vi "can_decoder2.vi"() -> ()   [LabVIEW 2015]
panel:
  out "tmp":dbl
  out "Waveform Chart 2":dynamicdata(graph)
  out "rate":dbl[](array[numeric]) format="%.2f"
  out "steering_torque":dbl format="%.2f"
  out "steering_angle":dbl format="%.2f"
  in  "IDs":u32[](array[numeric])=[0] format="%03x"
  in  "col size":i32
  in  "col idx":i32
  in  "ID":u32 format="%03x"
  out "Waveform Chart":dynamicdata(graph)
  in  "sortbyID":bool
  in  "clear":bool
  in  "sortbytime":bool
  out "can_log":u32[][](array[numeric]) format="%02x"
  out "error out":errorcluster
  # "Steering angle"
  # "Steering torque"
  # "RATE?"
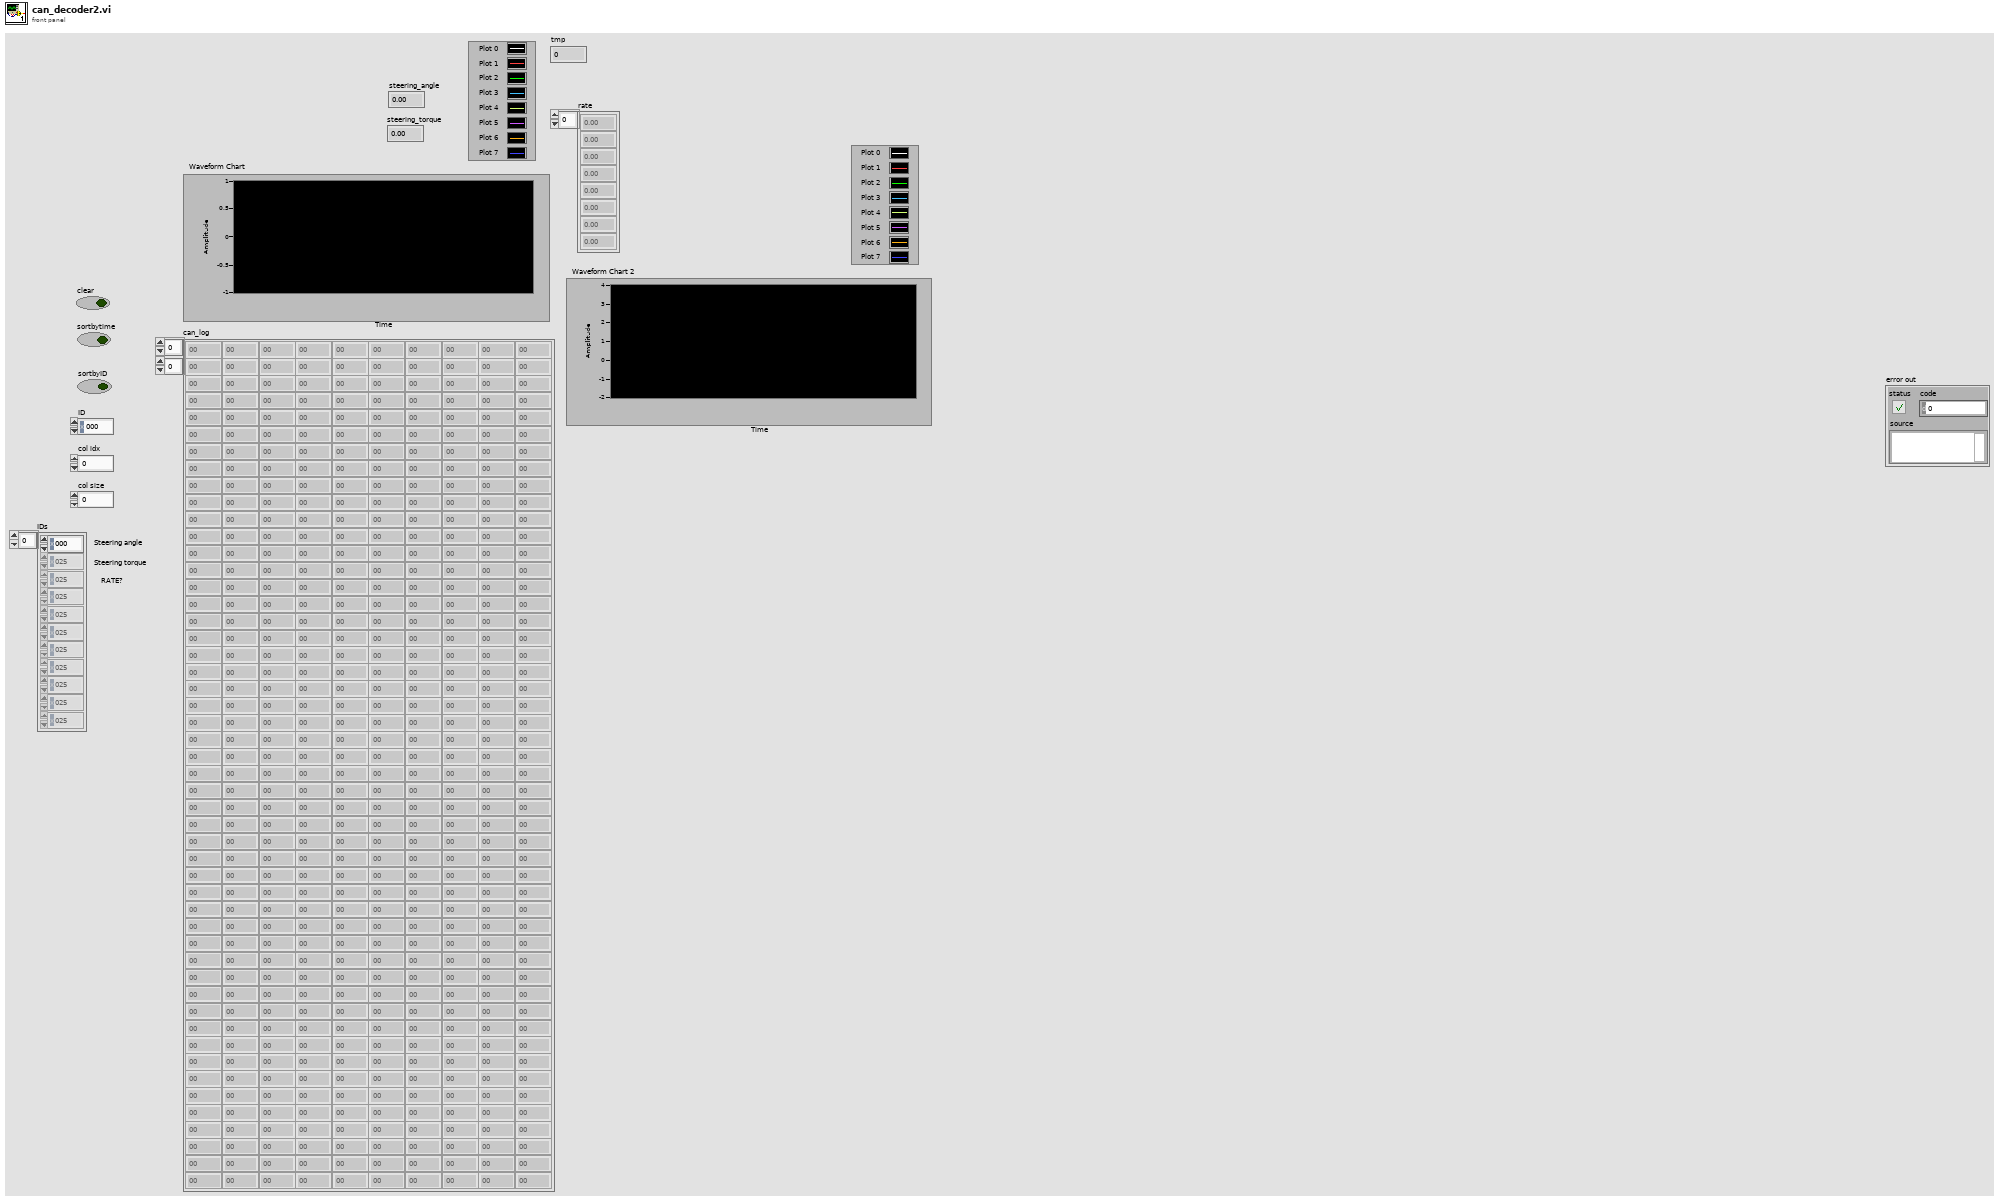
[diagram p1: front panel]
types:
  T1 = cluster{"Data[0]":u32, "Data[0]":u32, "Data[0]":u32, "Data[0]":u32, "Data[0]":u32, "Data[0]":u32, "Data[0]":u32, "Data[0]":u32, "Data[0]":u32, "Data[0]":u32, "Data[0]":u32}[]
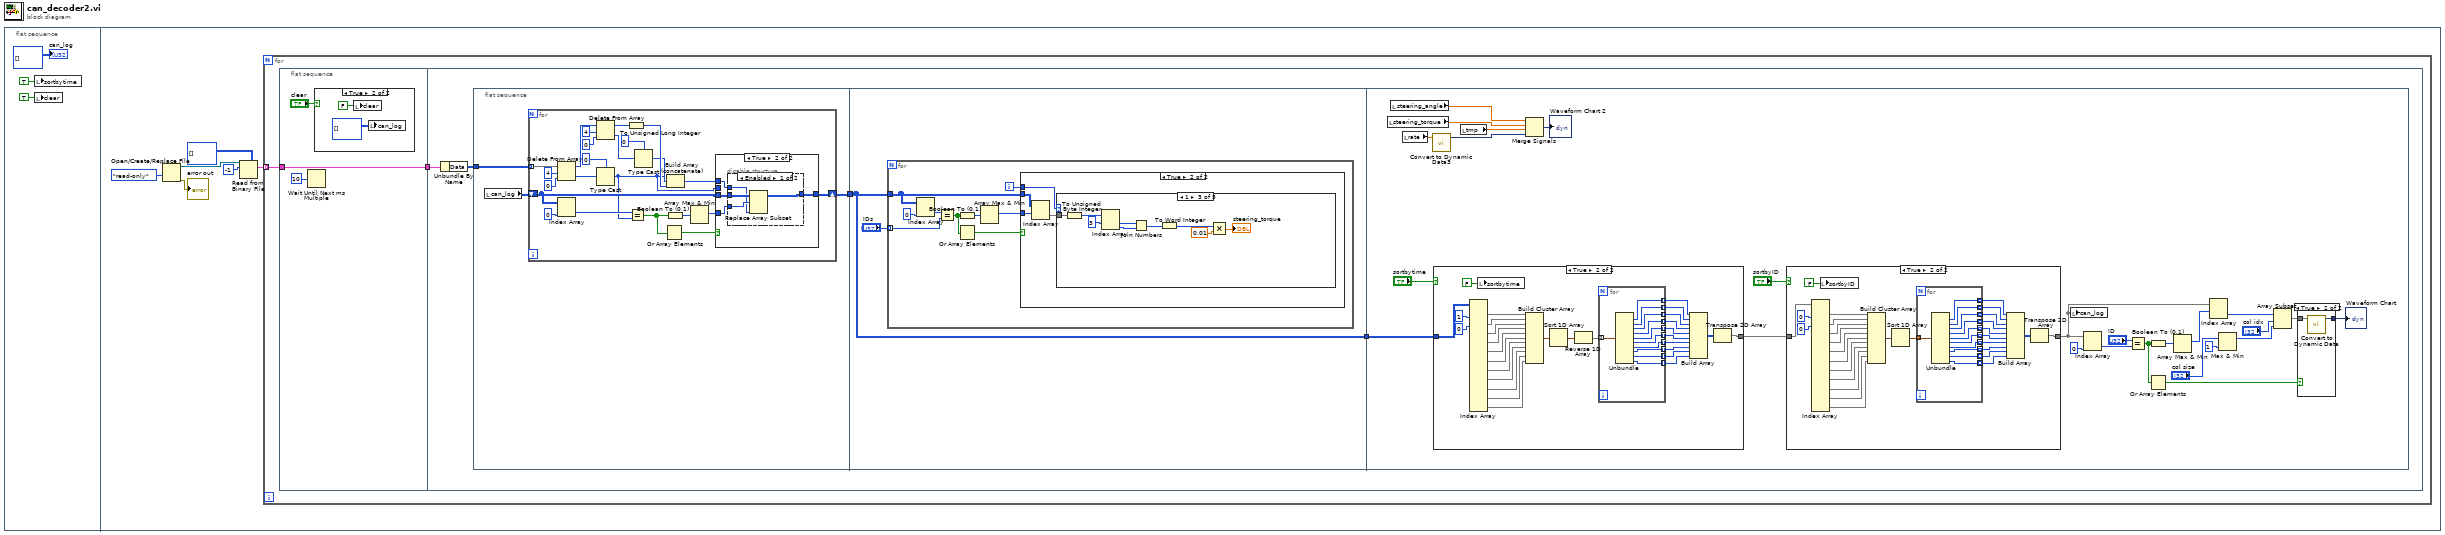
[diagram p0: block diagram]
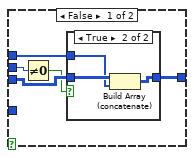
[diagram p3: hidden frame]
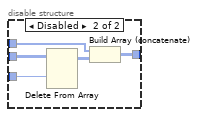
[diagram p5: hidden frame]
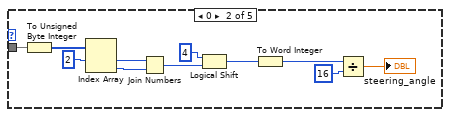
[diagram p8: hidden frame]
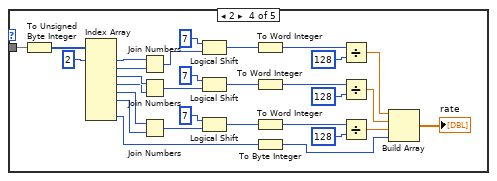
[diagram p9: hidden frame]
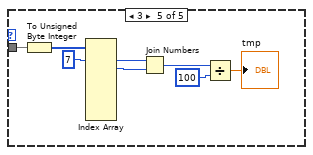
[diagram p10: hidden frame]
diagram:
  n1 = flat-sequence {
    frame #0 {
      n2 = local write "sortbytime"(TRUE ("sortbytime")) -> ()
      n3 = local write "clear"(TRUE ("clear")) -> ()
      "can_log" <- u32[][] [] ("can_log")
    }
    frame #1 {
      n4 = Open/Create/Replace File(access (0:read/write)=enum16{"read/write", "read-only", "write-only"}."read-only") -> (refnum out=w4:refnum<file>, error out=→"error out":errorcluster)  [unwired: 5 in, 1 out]
      n5 = Read from Binary File(5:u8[][] [] ("Data"), 10:-1 ("count (1)"), 11:w4) -> (2:w7:cluster{"Data":u8[][]}[])  [unwired: 3 in, 3 out]
      n6 = for {
        tunnel: w7 -> [w11] mode=indexing
        n7 = flat-sequence {
          tunnel: w11 -> [w14]
          tunnel: [w14] -> w10
          tunnel: w10 -> [w20]
          frame #0 {
            n8 = Wait Until Next ms Multiple(millisecond multiple=u32 10) -> ()  [unwired: 1 out]
            n9 = case shown="True" "clear" {
              frame False {
              }
              frame True {
                n10 = local write "clear"(FALSE ("clear")) -> ()
                n11 = local write "can_log"(u32[][] [] ("Data")) -> ()
              }
            }
          }
          frame #1 {
            n12 = Unbundle By Name(w20) -> ("Data"=w19:u8[][])
            n13 = flat-sequence {
              tunnel: w19 -> [w22]
              tunnel: [w21] -> w18
              tunnel: w18 -> [w69]
              tunnel: [w69] -> w17
              tunnel: w17 -> [w165]
              frame #0 {
                n14 = local read "can_log"() -> (w23:u32[][])
                n15 = for {
                  shift-right: [w29] -> w21
                  shift-left: w23 -> [w43]
                  tunnel: w22 -> [w38] mode=indexing
                  n16 = Delete From Array(array=w38, length=4, index=0) -> (deleted portion=w41:u8[], array with subset deleted=w35:u8[])
                  n17 = Index Array(array=w43, index (col)=0 ("disabled index (col)")) -> (element=w45:u32[])  [unwired: 1 in]
                  n18 = Delete From Array(array=w35, length=4, index=0) -> (deleted portion=w27:u8[], array with subset deleted=w34:u8[])
                  n19 = Type Cast(type=u32 0, x=w41) -> (*(type *) &x=w24:u32)
                  n20 = To Unsigned Long Integer(number=w34) -> (unsigned 32bit integer=w26:u32[])
                  n21 = Equal?(x=w45, y=w24) -> (x = y?=w32:bool[])
                  n22 = Type Cast(type=u32 0, x=w27) -> (*(type *) &x=w25:u32)
                  n23 = Or Array Elements(Boolean array=w32) -> (logical OR=w44:bool)
                  n24 = Boolean To (0,1)(Boolean=w32) -> (0, 1=w31:i16[])
                  n25 = Build Array (concatenate)(w24, w25, w26) -> (w33:u32[])
                  n26 = Array Max & Min(array=w31) -> (max index (indices)=w30:i32)  [unwired: 3 out]
                  n27 = case shown="True" w44 {
                    tunnel: w43 -> [w51 w59]
                    tunnel: [w50 w56] -> w29
                    tunnel: w33 -> [w49 w57]
                    tunnel: w30 -> [_ w58]
                    tunnel: w24 -> [w48 _]
                    frame False {
                      n28 = Not Equal To 0?(x=w48) -> (x != 0?=w47:bool)
                      n29 = case shown="True" w47 {
                        tunnel: w51 -> [w52 w55]
                        tunnel: [w52 w53] -> w50
                        tunnel: w49 -> [_ w54]
                        frame False {
                        }
                        frame True {
                          n30 = Build Array (concatenate)(w55, w54) -> (w53:u32[][])
                        }
                      }
                    }
                    frame True {
                      n31 = disable-structure shown="Enabled" {
                        disable-tunnel: w59 -> [w63 w68]
                        disable-tunnel: w58 -> [w62 w67]
                        disable-tunnel: w57 -> [w61 w65]
                        disable-tunnel: [w60 w64] -> w56
                        frame Enabled {
                          n32 = Replace Array Subset(array=w63, new element=w61, index (row)=w62) -> (w60:u32[][])  [unwired: 1 in]
                        }
                        frame Disabled {
                          n33 = Delete From Array(array=w68, index (row)=w67) -> (array with subset deleted=w66:u32[][])  [unwired: 2 in, 1 out]
                          n34 = Build Array (concatenate)(w65, w66) -> (w64:u32[][])
                        }
                      }
                    }
                  }
                }
              }
              frame #1 {
                n35 = for {
                  tunnel: "IDs" -> [w77] mode=indexing
                  tunnel: w69 -> [w72]
                  i -> [w71]
                  n36 = Index Array(array=w72, index (col)=0 ("disabled index (col)")) -> (element=w78:u32[])  [unwired: 1 in]
                  n37 = Equal?(x=w78, y=w77) -> (x = y?=w75:bool[])
                  n38 = Boolean To (0,1)(Boolean=w75) -> (0, 1=w76:i16[])
                  n39 = Or Array Elements(Boolean array=w75) -> (logical OR=w74:bool)
                  n40 = Array Max & Min(array=w76) -> (max index (indices)=w73:i32)  [unwired: 3 out]
                  n41 = case shown="True" w74 {
                    tunnel: w73 -> [_ w80]
                    tunnel: w72 -> [_ w83]
                    tunnel: w71 -> [_ w82]
                    frame False {
                    }
                    frame True {
                      n42 = Index Array(array=w83, index (row)=w80) -> (element=w81:u32[])  [unwired: 1 in]
                      n43 = case shown="1" w82 {
                        tunnel: w81 -> [_ w93 w102 w132 w139]
                        frame -1, Default {
                        }
                        frame 0 {
                          n44 = To Unsigned Byte Integer(number=w93) -> (unsigned 8bit integer=w92:u8[])
                          n45 = Index Array(array=w92, index #1=2 ("index")) -> (element #1=w91:u8, element #2=w90:u8)  [unwired: 1 in]
                          n46 = Join Numbers(hi=w91, lo=w90) -> ((hi.lo)=w89:u16)
                          n47 = Logical Shift(y=i16 4, x=w89) -> (x << y=w87:u16)
                          n48 = To Word Integer(number=w87) -> (16bit integer=w86:i16)
                          n49 = Divide(x=w86, y=i16 16) -> (x/y=→"steering_angle":dbl)
                        }
                        frame 1 {
                          n50 = To Unsigned Byte Integer(number=w102) -> (unsigned 8bit integer=w101:u8[])
                          n51 = Index Array(array=w101, index #1=3 ("index")) -> (element #1=w100:u8, element #2=w99:u8)  [unwired: 1 in]
                          n52 = Join Numbers(hi=w100, lo=w99) -> ((hi.lo)=w98:u16)
                          n53 = To Word Integer(number=w98) -> (16bit integer=w97:i16)
                          n54 = Multiply(x=w97, y=0.01) -> (x*y=→"steering_torque":dbl)
                        }
                        frame 2 {
                          n55 = To Unsigned Byte Integer(number=w132) -> (unsigned 8bit integer=w133:u8[])
                          n56 = Index Array(array=w133, index #1=2 ("index")) -> (element #1=w128:u8, element #2=w127:u8, element #3=w131:u8, element #4=w130:u8, element #5=w122:u8, element #6=w126:u8, element #8=w124:u8)  [unwired: 7 in, 1 out]
                          n57 = Join Numbers(hi=w128, lo=w127) -> ((hi.lo)=w114:u16)
                          n58 = Join Numbers(hi=w131, lo=w130) -> ((hi.lo)=w105:u16)
                          n59 = Join Numbers(hi=w122, lo=w126) -> ((hi.lo)=w118:u16)
                          n60 = Logical Shift(y=i16 7, x=w114) -> (x << y=w111:u16)
                          n61 = Logical Shift(y=i16 7, x=w105) -> (x << y=w109:u16)
                          n62 = Logical Shift(y=i16 7, x=w118) -> (x << y=w121:u16)
                          n63 = To Word Integer(number=w111) -> (16bit integer=w112:i16)
                          n64 = To Word Integer(number=w109) -> (16bit integer=w108:i16)
                          n65 = To Word Integer(number=w121) -> (16bit integer=w120:i16)
                          n66 = To Byte Integer(number=w124) -> (8bit integer=w123:i8)
                          n67 = Divide(x=w112, y=i16 128) -> (x/y=w110:dbl)
                          n68 = Divide(x=w108, y=i16 128) -> (x/y=w104:dbl)
                          n69 = Divide(x=w120, y=i16 128) -> (x/y=w117:dbl)
                          n70 = Build Array(w110, w104, w117, w123) -> (→"rate":dbl[])
                        }
                        frame 3 {
                          n71 = To Unsigned Byte Integer(number=w139) -> (unsigned 8bit integer=w141:u8[])
                          n72 = Index Array(array=w141, index #1=7 ("index")) -> (element #1=w138:u8, element #2=w137:u8)  [unwired: 7 in, 6 out]
                          n73 = Join Numbers(hi=w138, lo=w137) -> ((hi.lo)=w136:u16)
                          n74 = Divide(x=w136, y=u16 100) -> (x/y=→"tmp":dbl)
                        }
                      }
                    }
                  }
                }
              }
              frame #2 {
                n75 = local read "steering_torque"() -> (w145:dbl)
                n76 = local read "steering_angle"() -> (w146:dbl)
                n77 = local read "rate"() -> (w147:dbl[])
                n78 = call "Convert to Dynamic Data3"("Array"=w147) -> ("Dynamic Data Type"=w142:dynamicdata)  [unwired: 3 in]
                n79 = case shown="True" "sortbytime" {
                  tunnel: [w210 w212] -> w164
                  tunnel: w165 -> [w210 w240]
                  frame False {
                  }
                  frame True {
                    n80 = Index Array(array=w240, index (col) #1=1 ("disabled index (col)"), index (col) #2=0 ("index (col)")) -> (element #1=w237:u32[], element #2=w236:u32[], element #3=w235:u32[], element #4=w234:u32[], element #5=w233:u32[], element #6=w232:u32[], element #7=w231:u32[], element #8=w230:u32[], element #9=w229:u32[], element #10=w228:u32[], element #11=w227:u32[])  [unwired: 20 in]
                    n81 = local write "sortbytime"(FALSE ("sortbytime")) -> ()
                    n82 = Build Cluster Array(w237, w236, w235, w234, w233, w232, w231, w230, w229, w228, w227) -> (w226:T1)
                    n83 = Sort 1D Array(array=w226) -> (sorted array=w225:T1)
                    n84 = Reverse 1D Array(array=w225) -> (reversed array=w224:T1)
                    n85 = for {
                      tunnel: w224 -> [w251] mode=indexing
                      tunnel: [w250] -> w223 mode=indexing
                      tunnel: [w249] -> w222 mode=indexing
                      tunnel: [w248] -> w221 mode=indexing
                      tunnel: [w247] -> w220 mode=indexing
                      tunnel: [w246] -> w219 mode=indexing
                      tunnel: [w245] -> w218 mode=indexing
                      tunnel: [w244] -> w217 mode=indexing
                      tunnel: [w243] -> w216 mode=indexing
                      tunnel: [w242] -> w215 mode=indexing
                      tunnel: [w241] -> w214 mode=indexing
                      n86 = Unbundle(w251) -> ("Data[0]"=w250:u32, "Data[0]"=w249:u32, "Data[0]"=w248:u32, "Data[0]"=w247:u32, "Data[0]"=w246:u32, "Data[0]"=w245:u32, "Data[0]"=w244:u32, "Data[0]"=w243:u32, "Data[0]"=w242:u32, "Data[0]"=w241:u32)  [unwired: 1 out]
                    }
                    n87 = Build Array(w223, w222, w221, w220, w219, w218, w217, w216, w215, w214) -> (w213:u32[][])
                    n88 = Transpose 2D Array(2D array=w213) -> (transposed array=w212:u32[][])
                  }
                }
                n89 = local read "tmp"() -> (w143:dbl)
                n90 = Merge Signals(w146, w145, w143, w142) -> (→"Waveform Chart 2":dynamicdata)
                n91 = case shown="True" "sortbyID" {
                  tunnel: [w169 w172] -> w153
                  tunnel: w164 -> [w169 w198]
                  frame False {
                  }
                  frame True {
                    n92 = Index Array(array=w198, index (col) #1=0 ("disabled index (col)"), index (col) #2=0 ("index (col)")) -> (element #1=w195:u32[], element #2=w194:u32[], element #3=w193:u32[], element #4=w192:u32[], element #5=w191:u32[], element #6=w190:u32[], element #7=w189:u32[], element #8=w188:u32[], element #9=w187:u32[], element #10=w186:u32[], element #11=w185:u32[])  [unwired: 20 in]
                    n93 = local write "sortbyID"(FALSE ("sortbytime")) -> ()
                    n94 = Build Cluster Array(w195, w194, w193, w192, w191, w190, w189, w188, w187, w186, w185) -> (w184:T1)
                    n95 = Sort 1D Array(array=w184) -> (sorted array=w170:T1)
                    n96 = for {
                      tunnel: w170 -> [w209] mode=indexing
                      tunnel: [w208] -> w183 mode=indexing
                      tunnel: [w207] -> w182 mode=indexing
                      tunnel: [w206] -> w181 mode=indexing
                      tunnel: [w205] -> w180 mode=indexing
                      tunnel: [w204] -> w179 mode=indexing
                      tunnel: [w203] -> w178 mode=indexing
                      tunnel: [w202] -> w177 mode=indexing
                      tunnel: [w201] -> w176 mode=indexing
                      tunnel: [w200] -> w175 mode=indexing
                      tunnel: [w199] -> w174 mode=indexing
                      n97 = Unbundle(w209) -> ("Data[0]"=w208:u32, "Data[0]"=w207:u32, "Data[0]"=w206:u32, "Data[0]"=w205:u32, "Data[0]"=w204:u32, "Data[0]"=w203:u32, "Data[0]"=w202:u32, "Data[0]"=w201:u32, "Data[0]"=w200:u32, "Data[0]"=w199:u32)  [unwired: 1 out]
                    }
                    n98 = Build Array(w183, w182, w181, w180, w179, w178, w177, w176, w175, w174) -> (w173:u32[][])
                    n99 = Transpose 2D Array(2D array=w173) -> (transposed array=w172:u32[][])
                  }
                }
                n100 = local write "can_log"(w153) -> ()
                n101 = Index Array(array=w153, index (col)=0 ("disabled index (col)")) -> (element=w157:u32[])  [unwired: 1 in]
                n102 = Equal?(x="ID", y=w157) -> (x = y?=w159:bool[])
                n103 = Boolean To (0,1)(Boolean=w159) -> (0, 1=w158:i16[])
                n104 = Or Array Elements(Boolean array=w159) -> (logical OR=w160:bool)
                n105 = Array Max & Min(array=w158) -> (max index (indices)=w152:i32)  [unwired: 3 out]
                n106 = Index Array(array=w153, index (row)=w152) -> (element=w151:u32[])  [unwired: 1 in]
                n107 = Max & Min(x="col size", y=1) -> (max(x,y)=w149:i32)  [unwired: 1 out]
                n108 = Array Subset(array=w151, index="col idx", length=w149) -> (w156:u32[])
                n109 = case shown="True" w160 {
                  tunnel: w156 -> [_ w168]
                  tunnel: [_ w167] -> w148
                  frame False {
                  }
                  frame True {
                    n110 = call "Convert to Dynamic Data"("Array"=w168) -> ("Dynamic Data Type"=w167:dynamicdata)  [unwired: 3 in]
                  }
                }
                "Waveform Chart" <- w148
              }
            }
          }
        }
      }
    }
  }
